vi "제목없음 1.vi"() -> ()   [LabVIEW 2020]
uses:
  <vilib>/Utility/sysdir.llb/System Directory Type.ctl
panel:
  in  "채널 이름 입력(제목없음)":string[](array[string])
  in  "그룹 이름 입력(제목없음)":string
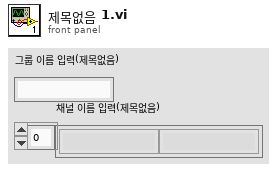
[diagram p1: front panel]
types:
  T1 = enum16{"open", "open or create", "create or replace", "create", "open (read-only)"}
  T2 = typedef "System Directory Type.ctl" = i32
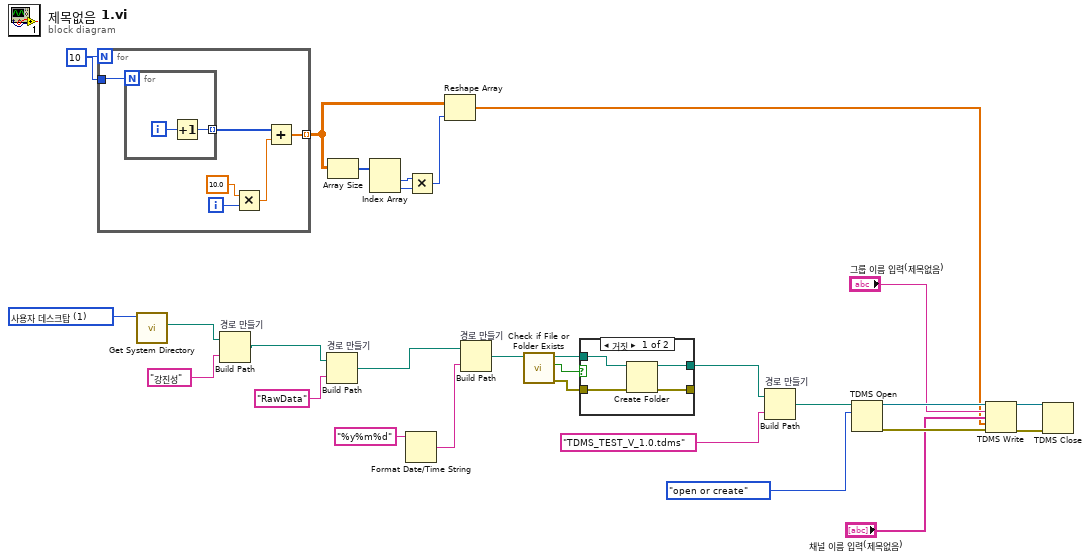
[diagram p0: block diagram]
diagram:
  w23 = T2 1 items=["사용자 홈"=0, "사용자 데스크탑"=1, "사용자 문서"=2, "사용자 어플리케이션 데이터"=3, "사용자 환경"=4, "사용자 임시"=5, "퍼블릭 문서"=6, "퍼블릭 어플리케이션 데이터"=7, "퍼블릭 환경"=8, "퍼블릭 캐시"=13, "시스템 코어 라이브러리"=9, "시스템 설치된 라이브러리"=10, "어플리케이션 파일"=11, "부팅 볼륨 루트"=12] ("system directory type")
  w29 = 10
  n1 = for {
    N: w29 -> [_]
    tunnel: w29 -> [w35]
    tunnel: [w30] -> w25 mode=indexing
    i -> [w33]
    n2 = for {
      N: w35 -> [_]
      tunnel: [w36] -> w32 mode=indexing
      i -> [w37]
      n3 = Increment(x=w37) -> (x+1=w36:i32)
    }
    n4 = Multiply(x=10.0, y=w33) -> (x*y=w31:dbl)
    n5 = Add(x=w32, y=w31) -> (x+y=w30:dbl[])
  }
  n6 = call <vilib>:"Get System Directory.vi"("system directory type"=w23) -> ("system directory"=w22:path)  [unwired: 10 in]
  n7 = Build Path "경로 만들기"(base path=w22, name or relative path="강진성") -> (appended path=w17:path)
  n8 = Build Path "경로 만들기"(base path=w17, name or relative path="RawData") -> (appended path=w16:path)
  n9 = Array Size(array=w25) -> (size(s)=w28:i32[])
  n10 = Index Array(array=w28) -> (element #1=w26:i32, element #2=w27:i32)  [unwired: 2 in]
  n11 = Format Date/Time String(time format string (%c)="%y%m%d" ("시간 포맷 문자열 (%c)")) -> (date/time string=w19:string)  [unwired: 2 in]
  n12 = Multiply(x=w26, y=w27) -> (x*y=w24:i32)
  n13 = Reshape Array(w25, w24) -> (w1:dbl[])
  n14 = Build Path "경로 만들기"(base path=w16, name or relative path=w19) -> (appended path=w15:path)
  n15 = call <vilib>:"Check if File or Folder Exists.vi"("path"=w15) -> ("error out"=w12:errorcluster, "file or folder exists?"=w14:bool, "dup path"=w13:path)  [unwired: 8 in]
  n16 = case shown="거짓" w14 {
    tunnel: w13 -> [w41 w43]
    tunnel: w12 -> [w40 w42]
    tunnel: [w39 w43] -> w11
    tunnel: [w38 w42] -> _
    frame False {
      n17 = Create Folder(path (use dialog)=w41, error in=w40) -> (created path=w39:path, error out=w38:errorcluster)  [unwired: 1 in, 1 out]
    }
    frame True {
    }
  }
  n18 = Build Path "경로 만들기"(base path=w11, name or relative path="TDMS_TEST_V_1.0.tdms") -> (appended path=w9:path)
  n19 = TDMS Open(10:T1."open or create" ("동작(0:open)"), 11:w9) -> (0:w6:errorcluster, 3:w7:refnum<k34>)  [unwired: 5 in]
  n20 = TDMS Write(0:w7, 5:"그룹 이름 입력(제목없음)", 7:"채널 이름 입력(제목없음)", 9:w1, 11:w6) -> (4:w3:refnum<k34>, 15:w2:errorcluster)  [unwired: 1 in, 2 out]
  n21 = TDMS Close(8:w2, 11:w3) -> ()  [unwired: 2 out]
